vi "Update Config Version.vi"(8 "error in (no error)":errorcluster, 10 "Cfg Version":string, 11 "NodeDiscovery in":refnum<class "DiscoveryService.lvclass">) -> (0 "error out":errorcluster, 3 "NodeDiscovery out":refnum<class "DiscoveryService.lvclass">)   [LabVIEW 2020, in "Vecto.lvlib" / "DiscoveryService.lvclass"]
uses:
  DiscoveryService.lvclass
  DiscoveryService.lvclass/DiscoveryService.ctl
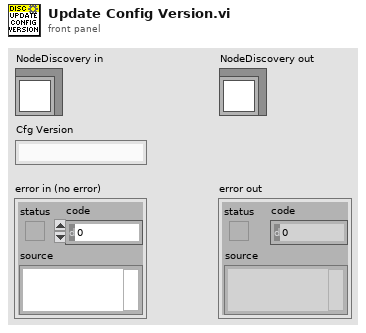
[diagram p1: front panel]
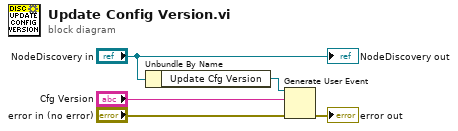
[diagram p0: block diagram]
diagram:
  n1 = Unbundle By Name("NodeDiscovery in") -> ("Update Cfg Version"=w4:refnum<user-event>)
  n2 = Generate User Event(user event=w4, event data cluster="Cfg Version", error in="error in (no error)") -> (error out=→"error out":errorcluster)  [unwired: 1 in, 1 out]
  "NodeDiscovery out" <- "NodeDiscovery in"
